vi "convertEncoderUnitsToCurrentUnits.vi"(8 "error in (no error)":errorcluster, 10 "Value In Encoder Units":dbl, 11 "Axis in":refnum<class "Axis.lvclass">) -> (0 "error out":errorcluster, 2 "Value In Current Units":dbl, 3 "Axis out":refnum<class "Axis.lvclass">)   [LabVIEW 2019, in "Axis.lvclass"]
uses:
  Axis.lvclass
  Axis.lvclass/Axis.ctl
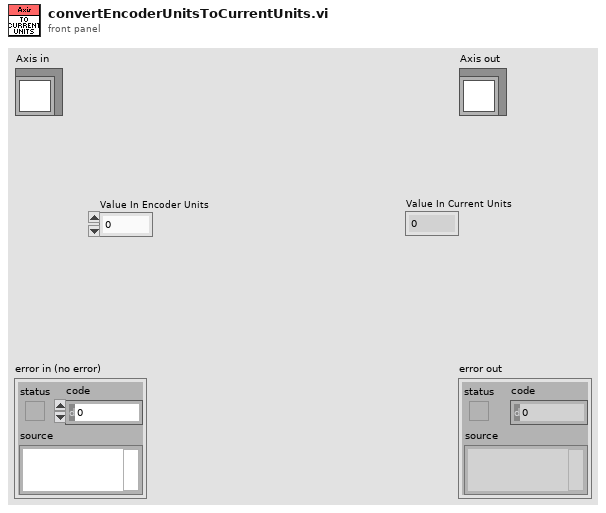
[diagram p1: front panel]
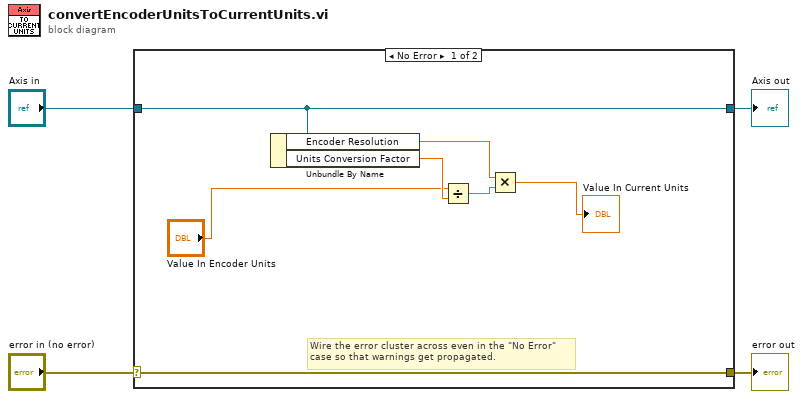
[diagram p0: block diagram]
diagram:
  n1 = case shown="No Error" "error in (no error)" {
    selector: "error in (no error)" -> [w11 w13]
    tunnel: [w11 w13] -> w3
    tunnel: [w10 w12] -> w1
    tunnel: "Axis in" -> [w10 w12]
    frame No Error {
      # "Wire the error cluster across even in the \"No Error\"\ncase so that warnings get propagated."
      n2 = Unbundle By Name(w10) -> ("Encoder Resolution"=w6:dbl, "Units Conversion Factor"=w9:dbl)
      n3 = Divide(x="Value In Encoder Units", y=w9) -> (x/y=w7:dbl)
      n4 = Multiply(x=w6, y=w7) -> (x*y=→"Value In Current Units":dbl)
    }
    frame Error {
    }
  }
  "error out" <- w3
  "Axis out" <- w1
